vi "float_to_real_4x1.vi"(10 "Float":dbl) -> (2 "REAL_4X1":string)   [LabVIEW 2018, in "Inficon IC6.lvlib"]
doc: "Format a float as an IC6 defined REAL_4X1 string."
uses:
  <instrlib>/Inficon IC6/Inficon IC6.lvlib
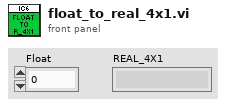
[diagram p1: front panel]
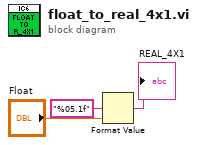
[diagram p0: block diagram]
diagram:
  n1 = Format Value(format string="%05.1f", value (0)="Float") -> (output string=→"REAL_4X1":string)  [unwired: 1 in]
